vi "initialise.vi"(8 "error in (no error)":errorcluster, 11 "ProEM_WinX32 in":refnum<class "ProEM_WinX32.lvclass">) -> (0 "error out":errorcluster, 3 "ProEM_WinX32 out":refnum<class "ProEM_WinX32.lvclass">)   [LabVIEW 2009, in "Hardware.lvlib" / "Channels.lvlib" / "ProEM_WinX32.lvclass"]
uses:
  ProEM_WinX32.lvclass
  ProEM_WinX32.lvclass/ProEM_WinX32.ctl
  Camera/Camera.lvclass
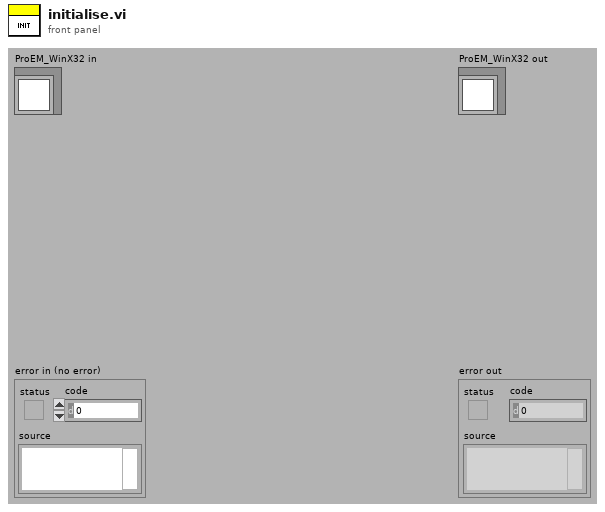
[diagram p1: front panel]
types:
  T1 = cluster{"Message":enum16{"Idle", "initialise", "configureAcquisition", "setTemperature", "getTemperature", "start", "stop", "sendImage", "close", "error", "ExitApp", "getAcquisitionStatus"}, "Data":variant}
  T2 = typedef "WINX32 Object Reference.ctl" = refnum<k1>
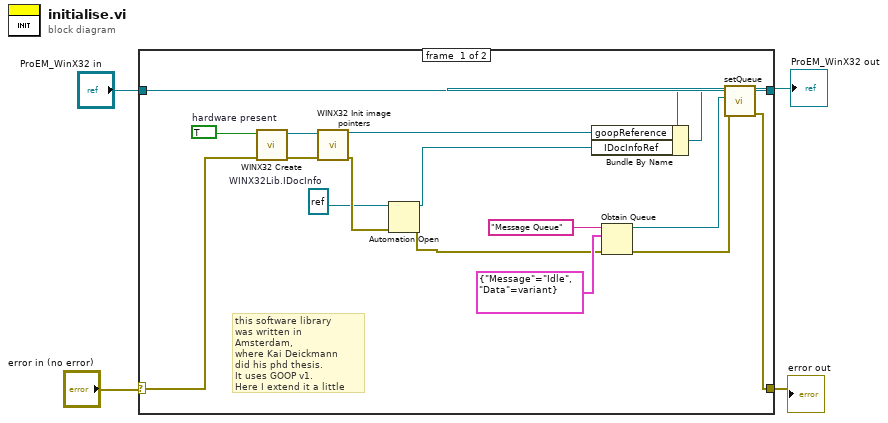
[diagram p0: block diagram]
diagram:
  n1 = case shown="No Error" "error in (no error)" {
    selector: "error in (no error)" -> [w20 w22]
    tunnel: [w8 w23] -> w4
    tunnel: "ProEM_WinX32 in" -> [w17 w23]
    tunnel: [w5 w22] -> w1
    frame #0 {
      w14 = refnum<k7> refnum  # WINX32Lib.IDocInfo
      w21 = TRUE  # hardware present
      # "this software library\nwas written in Amsterdam,\nwhere Kai Deickmann \ndid his phd thesis.\nIt uses GOOP v1.\nHere I extend it a little"
      n2 = call <instrlib>:"WINX32 Create.vi"("error in (no error)"=w20, "hardware present"=w21) -> ("error out"=w19:errorcluster, "reference"=w18:T2)  [unwired: 4 in]
      n3 = call <instrlib>:"WINX32 Init image pointers.vi"("error in (no error)"=w19, "reference"=w18) -> ("error out"=w15:errorcluster, "duplicate reference"=w16:T2)  [unwired: 8 in]
      n4 = Automation Open(error in (no error)=w15, Automation Refnum=w14) -> (Automation Refnum=w13:refnum<k7>, error out=w10:errorcluster)  [unwired: 2 in]
      n5 = Bundle By Name(cluster=w17, "goopReference"=w16, "IDocInfoRef"=w13) -> (w9:refnum<class "ProEM_WinX32.lvclass">)
      n6 = Obtain Queue(name (unnamed)="Message Queue" ("Queue Name"), element data type=T1 {"Message"=enum."Idle", "Data"=variant}, error in (no error)=w10) -> (queue out=w7:refnum<queue>, error out=w6:errorcluster)  [unwired: 2 in, 1 out]
      n7 = call "setQueue.vi"("error in (no error)"=w6, "queue"=w7, "Camera in"=w9) -> ("error out"=w5:errorcluster, "Camera out"=w8:refnum<class "ProEM_WinX32.lvclass">)  [unwired: 7 in]
    }
    frame #1 {
    }
  }
  "error out" <- w1
  "ProEM_WinX32 out" <- w4
